vi "Mouse Up.vi"(8 "error in (no error)":errorcluster, 9 "button info":T2, 10 "axis info":T1, 11 "UI_Top_Customer in":refnum<class "UI_Top_Customer.lvclass">) -> (0 "error out":errorcluster, 3 "UI_Top_Customer out":refnum<class "UI_Top_Customer.lvclass">)   [LabVIEW 2021, in "UI_Top_Customer.lvclass"]
uses:
  UI_Top_Customer.lvclass
  UI_Top_Customer.lvclass/UI_Top_Customer.ctl
  <vilib>/ptbypt/NI_PtbyPt.lvlib
  <userlib>/John_Lib/AbstractActorTemplate/UIActorTop Messages/UI Initialize Msg/UI Initialize Msg.lvclass
  <vilib>/ActorFramework/Actor/Actor.lvclass
  C:/Program Files (x86)/National Instruments/LabVIEW 2021/user.lib/John_Lib/AbstractActorTemplate/AbstractActorTemplate/UIActorTop.lvclass
  C:/Program Files (x86)/National Instruments/LabVIEW 2021/vi.lib/ActorFramework/Actor/Actor.lvclass
  C:/Program Files (x86)/National Instruments/LabVIEW 2021/project/Create Actor from Template/_UI_Top_Customer/UI_Top_Customer.lvclass
  C:/Program Files (x86)/National Instruments/LabVIEW 2021/user.lib/John_Lib/Interfaces/FrontPanel Save Image/FrontPanel Save Image.lvclass
  C:/Program Files (x86)/National Instruments/LabVIEW 2021/user.lib/John_Lib/Interfaces/InsertMainSubPanel/InsertMainSubPanel.lvclass
panel:
  out "current time":timestamp
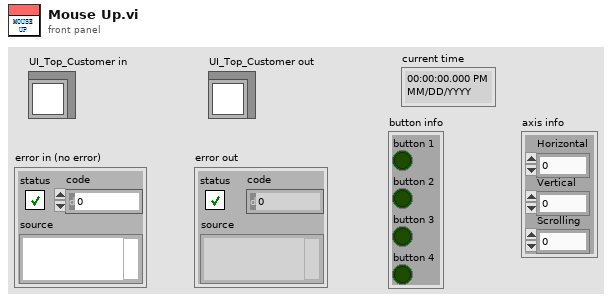
[diagram p1: front panel]
types:
  T1 = cluster{"Horizontal":i32, "Vertical":i32, "Scrolling":i32}
  T2 = cluster{"button 1":bool, "button 2":bool, "button 3":bool, "button 4":bool}
  T3 = enum32{"Invalid", "Standard", "Closed", "Hidden", "Minimized", "Maximized"}
  T4 = typedef "UI_Top_Customer.lvlib/UI_Top_Customer.lvclass/Pane MouseDown.ctl" = cluster{"Type":T5, "Coords":T6, "Mods":cluster{"Double Click":bool, "Menu Key":bool}, "Pane: MouseDown":bool}
  T5 = typedef "lveventtype.ctl" = enum32{"Null", "Timeout", "Annotation Menu Selection", "Annotation Menu Selection?", "App Instance Close", "App Instance Close?", "Autoscale Range Change", "Bookmark Info Change", "Cell Edit", "Cell Edit?", "Cursor Grab", "Cursor Grab?", "Cursor Menu Selection", "Cursor Menu Selection?", "Cursor Move", "Cursor Release", "Data Change", "Direction Change", "Display State Change", "Drag Ended", "Drag Enter", "Drag Leave", "Drag Over", "Drag Source Update", "Drag Starting", "Drag Starting?", "Drop", "Exec State Change", "Key Down", "Key Down?", "Key Repeat", "Key Repeat?", "Key Up", "Listbox Double Click", "Menu Activation?", "Menu Selection (App)", "Menu Selection? (App)", "Menu Selection (User)", "Mouse Down", "Mouse Down?", "Mouse Enter", "Mouse Leave", "Mouse Move", "Mouse Up", "Mouse Wheel", "NI Security User Change (App)", "Pane Size", "Panel Close", "Panel Close?", "Panel Resize", "Plot Attribute Change", "Scale Range Change", "Shortcut Menu Activation?", "Shortcut Menu Selection (App)", "Shortcut Menu Selection? (App)", "Shortcut Menu Selection (User)", "Tree Double Click", "Tree Drag", "Tree Drag?", "Tree Drop", "Tree Drop?", "Tree Item Close", "Tree Item Close?", "Tree Item Open", "Tree Item Open?", "User Event", "Value Change"}
  T6 = typedef "LVPoint32TypeDef.ctl" = cluster{"Horizontal":i32, "Vertical":i32}
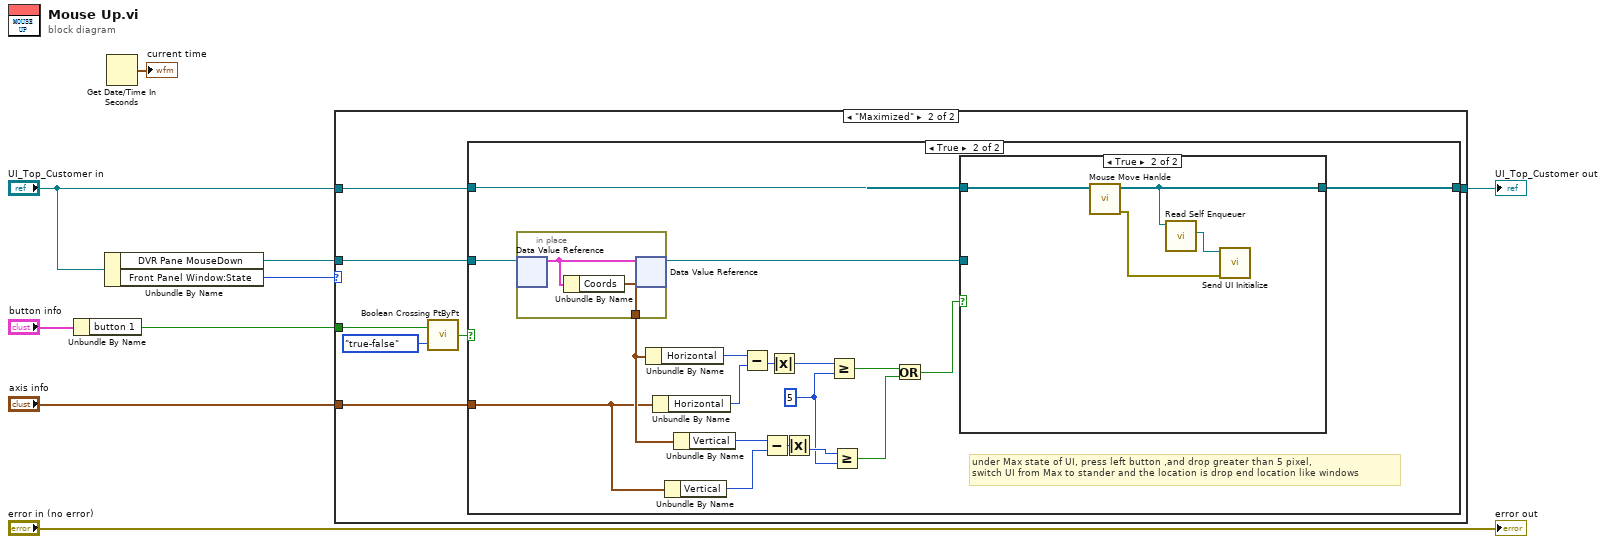
[diagram p0: block diagram]
diagram:
  n1 = Unbundle By Name("button info") -> ("button 1"=w5:bool)
  n2 = Unbundle By Name("UI_Top_Customer in") -> ("DVR Pane MouseDown"=w1:refnum<data-value>, "Front Panel Window:State"=w8:T3)
  n3 = Get Date/Time In Seconds() -> (seconds since 1Jan1904=→"current time":timestamp)
  n4 = case shown="\"Maximized\"" w8 {
    tunnel: "UI_Top_Customer in" -> [w10 w14]
    tunnel: [w10 w13] -> w7
    tunnel: w5 -> [_ w17]
    tunnel: "axis info" -> [_ w11]
    tunnel: w1 -> [_ w12]
    frame "Invalid", Default {
    }
    frame "Maximized" {
      n5 = call <vilib>:"Boolean Crossing PtByPt.vi"("direction"=enum16{"either", "false-true", "true-false"}."true-false", "input"=w17) -> ("crossing"=w15:bool)  [unwired: 1 in]
      n6 = case shown="True" w15 {
        tunnel: w14 -> [w18 w20]
        tunnel: [w18 w19] -> w13
        tunnel: w12 -> [_ w36]
        tunnel: w11 -> [_ w30]
        frame False {
        }
        frame True {
          w21 = 5 ("y")
          # "under Max state of UI, press left button ,and drop greater than 5 pixel, \nswitch UI from Max to stander and the location is drop end location like windows"
          n7 = in-place {
            in-place-border: [w42] -> w31
            n8 = in-place-dvr #1(w36) -> (w43:T4)  [unwired: 1 out]
            n9 = Unbundle By Name(w43) -> ("Coords"=w42:T6)
            n10 = in-place-dvr #1(w43) -> (w25:refnum<data-value>)  [unwired: 1 out]
          }
          n11 = Unbundle By Name(w31) -> ("Horizontal"=w35:i32)
          n12 = Unbundle By Name(w30) -> ("Horizontal"=w34:i32)
          n13 = Unbundle By Name(w30) -> ("Vertical"=w33:i32)
          n14 = Unbundle By Name(w31) -> ("Vertical"=w32:i32)
          n15 = Subtract(x=w35, y=w34) -> (x-y=w29:i32)
          n16 = Subtract(x=w32, y=w33) -> (x-y=w28:i32)
          n17 = Absolute Value(x=w29) -> (abs(x)=w23:i32)
          n18 = Absolute Value(x=w28) -> (abs(x)=w22:i32)
          n19 = Greater Or Equal?(x=w23, y=w21) -> (x >= y?=w27:bool)
          n20 = Greater Or Equal?(x=w22, y=w21) -> (x >= y?=w26:bool)
          n21 = Or(x=w27, y=w26) -> (x .or. y?=w24:bool)
          n22 = case shown="True" w24 {
            tunnel: w25 -> [_ _]
            tunnel: w20 -> [w37 w41]
            tunnel: [w37 w39] -> w19
            frame False {
            }
            frame True {
              n23 = call "Mouse Move Hanlde.vi"("UI_Top_Customer in"=w41) -> ("error out"=w40:errorcluster, "UI_Top_Customer out"=w39:refnum<class "UI_Top_Customer.lvclass">)  [unwired: 9 in]
              n24 = call <vilib>:"Read Self Enqueuer.vi"("Actor"=w39) -> ("Self Enqueuer"=w38:refnum<class "Message Enqueuer.lvclass">)  [unwired: 10 in]
              n25 = call <userlib>:"Send UI Initialize.vi"("error in (no error)"=w40, "Message Enqueuer"=w38) -> ()  [unwired: 8 in, 2 out]
            }
          }
        }
      }
    }
  }
  "UI_Top_Customer out" <- w7
  "error out" <- "error in (no error)"
